vi "to_utc.vi"(1 "Numeric":dbl) -> (0 "Time Stamp":timestamp)   [LabVIEW 2010]
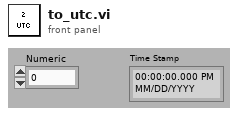
[diagram p1: front panel]
types:
  T1 = typedef "LVDateTimeRec.ctl" = cluster{"fractional second":dbl, "second":i32, "minute":i32, "hour":i32, "day of month":i32, "month":i32, "year":i32, "day of week":i32, "day of year":i32, "DST":i32}
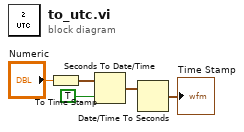
[diagram p0: block diagram]
diagram:
  n1 = To Time Stamp(1:"Numeric") -> (0:w1:timestamp)
  n2 = Seconds To Date/Time(time stamp (now)=w1, to UTC (F)=TRUE) -> (date time rec=w4:T1)
  n3 = Date/Time To Seconds(2:w4) -> (0:→"Time Stamp":timestamp)  [unwired: 1 in]
